vi "Queue FGV.vi"(8 "error in":errorcluster, 9 "Queue name (unnamed)":string, 10 "Queue Action":T1) -> (0 "error out":errorcluster, 3 "Queue reference":refnum<queue>)   [LabVIEW 2018, in "Covers-o-meter.lvlib"]
doc: "FGV to create/get/destroy user event. User event is used to stop all modules."
uses:
  Covers-o-meter.lvlib
  ctl/Queue action--enum.ctl
  ctl/Message--enum.ctl
  ctl/State--enum.ctl
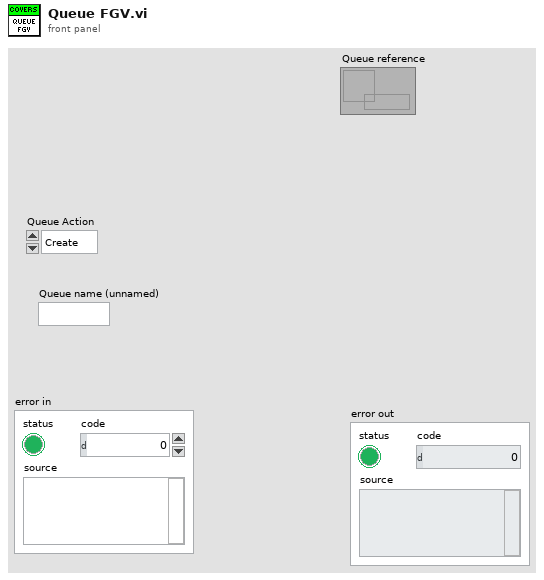
[diagram p1: front panel]
types:
  T1 = typedef "Covers-o-meter.lvlib/Queue action--enum.ctl" = enum16{"Create", "Get", "Destroy"}
  T2 = typedef "Covers-o-meter.lvlib/Message--enum.ctl" = cluster{"State":T3, "Data":variant}
  T3 = typedef "Covers-o-meter.lvlib/State--enum.ctl" = enum16{"Init", "Init: Read req tags", "Init Data: All Projects", "Init: Which Project?", "Update Requirements tags", "Get all project strings", "Search proj for tags", "Subroutine", "Update Project", "Start Button Pressed", "Start timer", "Error", "Close", "UI - Refresh Timer ", "UI - refresh graph", "UI - Refresh Tree"}
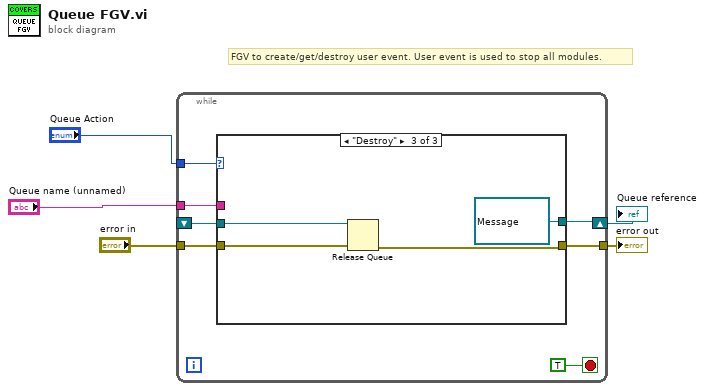
[diagram p0: block diagram]
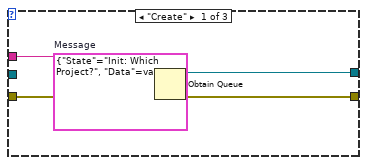
[diagram p2: hidden frame]
diagram:
  # "FGV to create/get/destroy user event. User event is used to stop all modules."
  n1 = while {
    tunnel: "Queue Action" -> [w11]
    shift-right: [w10] -> w1
    shift-left: _ -> [w9]
    tunnel: [w8] -> w5
    tunnel: "error in" -> [w7]
    tunnel: "Queue name (unnamed)" -> [w6]
    stop <- TRUE stop-if-true
    n2 = case shown="\"Destroy\"" w11 {
      tunnel: [w17 w19 refnum<queue> refnum ("queue out")] -> w10
      tunnel: w9 -> [_ w19 w23]
      tunnel: [w16 w18 w21] -> w8
      tunnel: w7 -> [w15 w18 w22]
      tunnel: w6 -> [w14 _ _]
      frame "Create" {
        w13 = T2 {"State"=enum."Init: Which Project?", "Data"=variant}  # Message
        n3 = Obtain Queue(name (unnamed)=w14, element data type=w13, error in (no error)=w15) -> (queue out=w17:refnum<queue>, error out=w16:errorcluster)  [unwired: 2 in, 1 out]
      }
      frame "Get", Default {
      }
      frame "Destroy" {
        n4 = Release Queue(queue=w23, error in (no error)=w22) -> (error out=w21:errorcluster)  [unwired: 1 in, 2 out]
      }
    }
  }
  "error out" <- w5
  "Queue reference" <- w1
